vi "Wait for Acquisition Complete.vi"(8 "error in (no error)":errorcluster, 9 "Maximum Time (10000)":u32=10000, 11 "VISA resource name":refnum<visa-resource-name>) -> (0 "error out":errorcluster, 3 "VISA resource name out":refnum<visa-resource-name>)   [LabVIEW 2020, in "Template - Spectrum Analyzer.lvlib"]
doc: "Waits for the current sweep to finish. This VI should be called after <b>Initiate</b> VI and before <b>Fetch Trace</b> VI.\n\n<B>Note:</B> \n\nUse this VI only with other low-level VIs. The high-level VIs automatically incorporate this functionality. This VI does not check the instrument status."
uses:
  <instrlib>/_Template - Spectrum Analyzer/Template - Spectrum Analyzer.lvlib
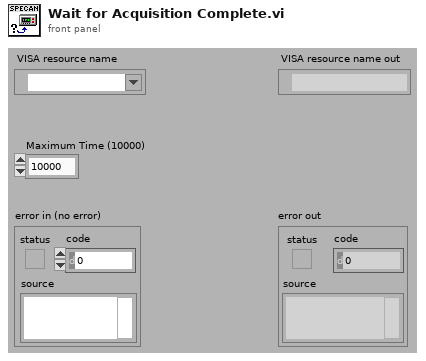
[diagram p1: front panel]
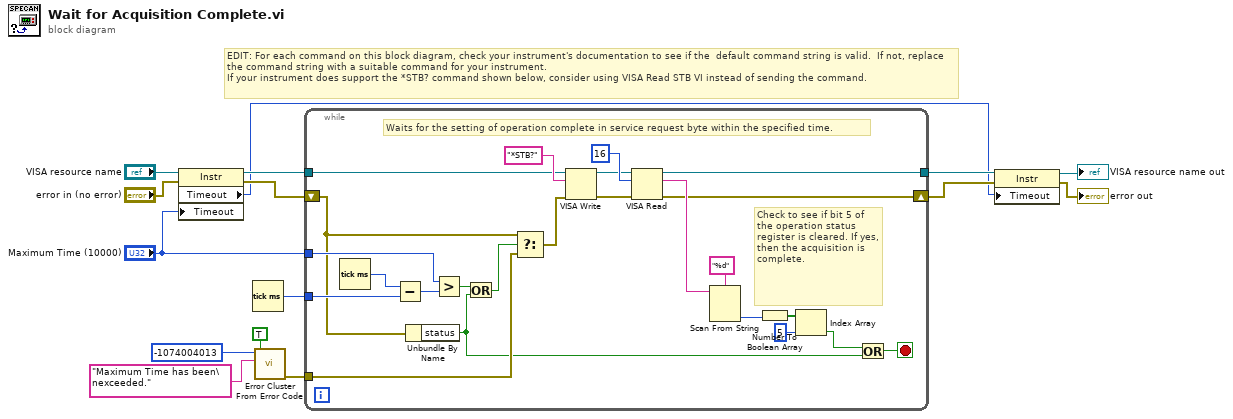
[diagram p0: block diagram]
diagram:
  # "EDIT: For each command on this block diagram, check your instrument's documentation to see if the  default command string is valid.  If not, replace the command string with a suitable command for your instrument. \nIf your instrument does support the *STB? command shown below, consider using VISA Read STB VI instead of sending the command."
  n1 = property class="Instr"(reference="VISA resource name", error in="error in (no error)", "Timeout"="Maximum Time (10000)") -> (reference out=w3:refnum<visa-resource-name>, error out=w2:errorcluster, "Timeout"=w1:u32)
  n2 = Tick Count (ms)() -> (millisecond timer value=w15:u32)
  n3 = call <vilib>:"Error Cluster From Error Code.vi"("show call chain? (False)"=TRUE, "error message (\"\")"="Maximum Time has been\nexceeded." ("error message (\"\")"), "error code (0)"=-1074004013) -> ("error out"=w11:errorcluster)  [unwired: 6 in]
  n4 = while {
    tunnel: [w36] -> w9
    tunnel: w3 -> [w33]
    tunnel: "Maximum Time (10000)" -> [w27]
    tunnel: w15 -> [w28]
    shift-right: [w37] -> w10
    shift-left: w2 -> [w20]
    tunnel: w11 -> [w18]
    stop <- w23 stop-if-true
    # "Waits for the setting of operation complete in service request byte within the specified time."
    # "Check to see if bit 5 of the operation status register is cleared. If yes, then the acquisition is complete."
    n5 = Tick Count (ms)() -> (millisecond timer value=w30:u32)
    n6 = Subtract(x=w30, y=w28) -> (x-y=w29:u32)
    n7 = Unbundle By Name(w20) -> ("status"=w16:bool)
    n8 = Greater?(x=w27, y=w29) -> (0:w17:bool)
    n9 = Or(x=w17, y=w16) -> (x .or. y?=w21:bool)
    n10 = Select(t=w20, s=w21, f=w18) -> (s? t:f=w19:errorcluster)
    n11 = VISA Write(VISA resource name=w33, write buffer="*STB?", error in (no error)=w19) -> (VISA resource name out=w31:refnum<visa-resource-name>, error out=w32:errorcluster)  [unwired: 1 out]
    n12 = VISA Read(VISA resource name=w31, byte count=u32 16, error in (no error)=w32) -> (VISA resource name out=w36:refnum<visa-resource-name>, read buffer=w39:string, error out=w37:errorcluster)  [unwired: 1 out]
    n13 = Scan From String(format string="%d", input string=w39) -> (output 1=w25:i32)  [unwired: 3 in, 3 out]
    n14 = Number To Boolean Array(number=w25) -> (Boolean array=w24:bool[])
    n15 = Index Array(array=w24, index=5) -> (element=w22:bool)
    n16 = Or(x=w22, y=w16) -> (x .or. y?=w23:bool)
  }
  n17 = property class="Instr"(reference=w9, error in=w10, "Timeout"=w1) -> (reference out=→"VISA resource name out":refnum<visa-resource-name>, error out=→"error out":errorcluster)
